vi "Drive Train Temps.vi"(8 "error in (no error)":errorcluster, 10 "Force Throttle?":bool, 11 "Falcon500 in":refnum<class "Falcon500.lvclass">) -> (0 "error out":errorcluster, 2 "Drive Train Tempuratures":T1, 3 "Falcon500 out":refnum<class "Falcon500.lvclass">)   [LabVIEW 2019, in "Drive.lvlib" / "Falcon500.lvclass"]
uses:
  Falcon500.lvclass
  C:/Users/Public/Documents/2020InfinteRecharge/src robot/Classes/Drive/Tank Drive/Tank Drive.lvclass
  Controls/Drive Train Temperatures.ctl
  <vilib>/Rock Robotics/WPI/ThirdParty/Phoenix-LabVIEW/Motor Controller/Controls/CTRE_Phoenix_MotorControl_StatorCurrentLimitConfiguration.ctl
  <vilib>/Rock Robotics/WPI/ThirdParty/Phoenix-LabVIEW/Motor Controller/Get/CTRE_Phoenix_MotorController_GetTemperature.vi
  <vilib>/Rock Robotics/Network Tables/NT Write Boolean.vi
  CTRE Drive.lvclass
  Tank Drive.lvclass
panel:
  out "Throttle?":bool
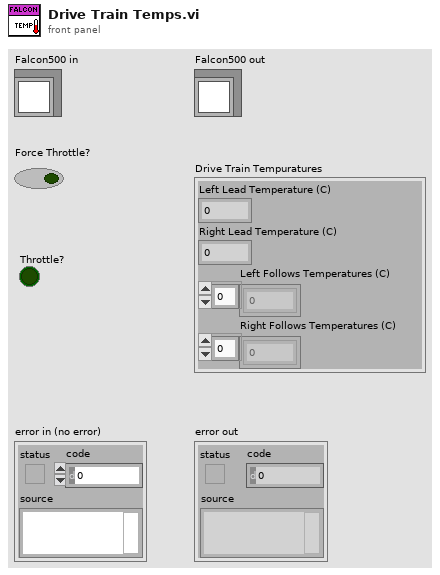
[diagram p1: front panel]
types:
  T1 = typedef "Drive.lvlib/Tank Drive.lvclass/Drive Train Temperatures.ctl" = cluster{"Left Lead Temperature (C)":dbl, "Right Lead Temperature (C)":dbl, "Left Follows Temperatures (C)":dbl[], "Right Follows Temperatures (C)":dbl[]}
  T2 = typedef "CTRE_Phoenix_MotorControl_StatorCurrentLimitConfiguration.ctl" = cluster{"Enable?":bool, "Current Limit":dbl, "Threshold Current":dbl, "Threshold Time":dbl}
  T3 = typedef "Drive.lvlib/Tank Drive.lvclass/Motor Controller Names.ctl" = cluster{"Left Lead":string, "Right Lead":string, "Left Followers":string[], "Right Followers":string[]}
  T4 = typedef "WPI_MotorControlDeviceRef.ctl" = cluster{"DeviceStatus":errorcluster, "Type":T5, "PWM":cluster{"PWM Channel":T6, "DeadBand":T7}, "CAN":cluster{"Device Number":u8, "SetOutput VI Ref":variant, "GetOutput VI Ref":variant, "Enable VI Ref":variant, "Disable VI Ref":variant, "Data":variant}, "Invert":bool, "DIO PWM":cluster{"PWM \"Enable\" Channel":T6, "DIOChannel":T8, "PWM Rate":dbl}}
  T5 = typedef "WPI_MotorControlType.ctl" = enum16{"PWM", "CAN", "DIO PWM"}
  T6 = typedef "FPGA_DIOPWMChannel.ctl" = enum8{"PWM 0", "PWM 1", "PWM 2", "PWM 3", "PWM 4", "PWM 5", "PWM 6", "PWM 7", "PWM 8", "PWM 9", "PWM MXP 0", "PWM MXP 1", "PWM MXP 2", "PWM MXP 3", "PWM MXP 4", "PWM MXP 5", "PWM MXP 6", "PWM MXP 7", "PWM MXP 8", "PWM MXP 9", "Invalid"}
  T7 = typedef "WPI_PWMDeadband.ctl" = cluster{"Name":string, "maxPositivePwm":i32, "minPositivePwm":i32, "centerPwm":i32, "maxNegativePwm":i32, "minNegativePwm":i32, "angularRange":u16}
  T8 = typedef "FPGA_DIOChannel.ctl" = enum8{"DIO 0", "DIO 1", "DIO 2", "DIO 3", "DIO 4", "DIO 5", "DIO 6", "DIO 7", "DIO 8", "DIO 9", "DIO MXP 0", "DIO MXP 1", "DIO MXP 2", "DIO MXP 3", "DIO MXP 4", "DIO MXP 5", "DIO MXP 6", "DIO MXP 7", "DIO MXP 8", "DIO MXP 9", "DIO MXP 10", "DIO MXP 11", "DIO MXP 12", "DIO MXP 13", "DIO MXP 14", "DIO MXP 15", "SPI Port CS1", "SPI Port CS2", "SPI Port CS3", "SPI Port MISO", "SPI Port MOSI", "Invalid"}
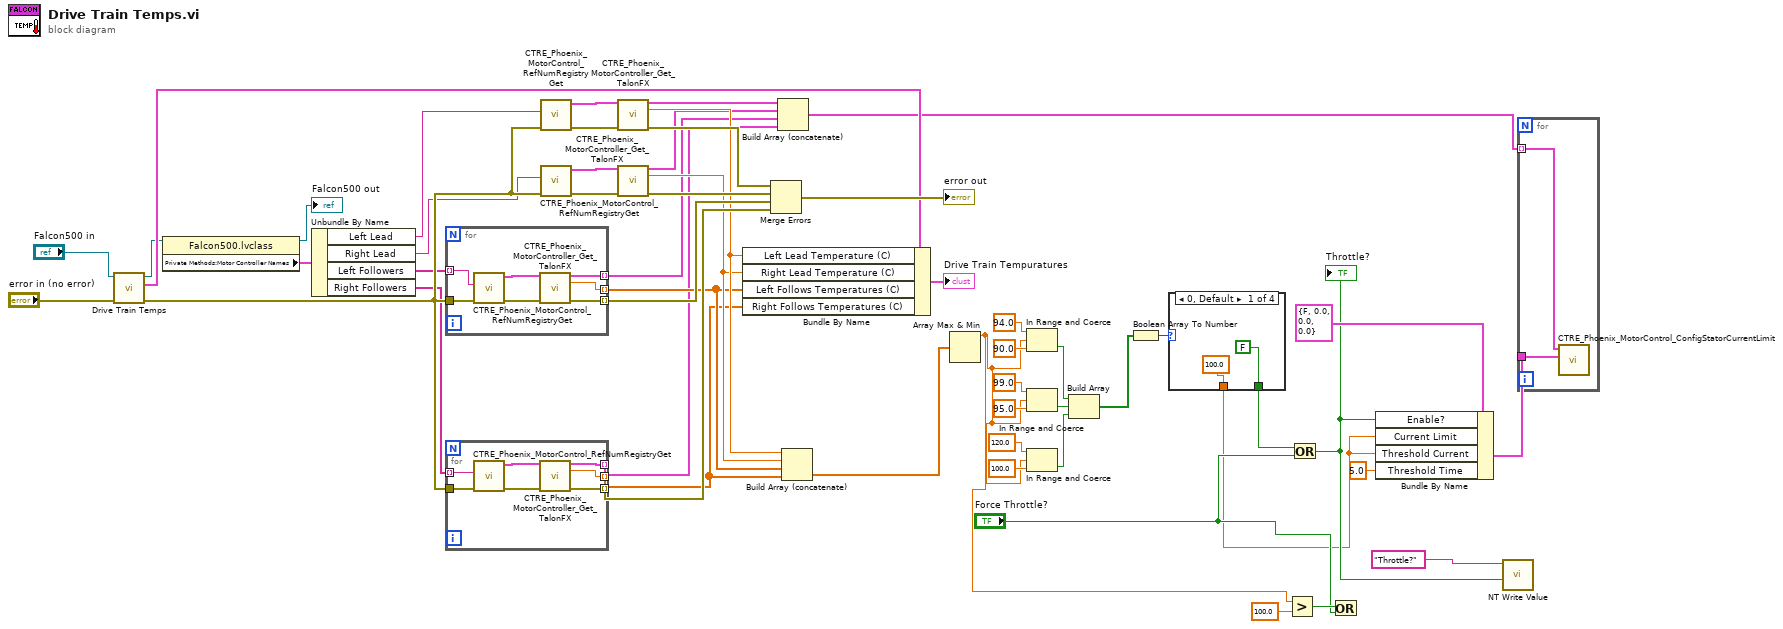
[diagram p0: block diagram]
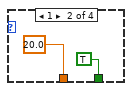
[diagram p2: hidden frame]
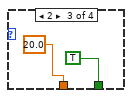
[diagram p3: hidden frame]
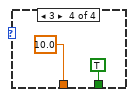
[diagram p4: hidden frame]
diagram:
  n1 = call-parent "Drive Train Temps.vi"("error in (no error)"="error in (no error)", "Tank Drive in"="Falcon500 in") -> ("error out"=w40:errorcluster, "Drive Train Temperatures"=w34:T1, "Tank Drive out"=w33:refnum<class "Falcon500.lvclass">)  [unwired: 7 in]
  n2 = property class="Falcon500.lvclass"(reference=w33) -> (reference out=→"Falcon500 out":refnum<class "Falcon500.lvclass">, "Private Methods:Motor Controller Names"=w52:T3)  [unwired: 1 in, 1 out]
  n3 = Unbundle By Name(w52) -> ("Left Lead"=w30:string, "Right Lead"=w29:string, "Left Followers"=w28:string[], "Right Followers"=w27:string[])
  n4 = for {
    tunnel: w28 -> [w58] mode=indexing
    tunnel: [w57] -> w37 mode=indexing
    tunnel: [w56] -> w44 mode=indexing
    tunnel: w40 -> [w55]
    tunnel: [w54] -> w22 mode=indexing
    n5 = call <vilib>:"CTRE_Phoenix_MotorControl_RefNumRegistryGet.vi"("error in (no error)"=w55, "refnum name"=w58) -> ("error out"=w59:errorcluster, "PhoenixMotorControlDevRef"=w60:T4)  [unwired: 8 in]
    n6 = call-poly <vilib>:"CTRE_Phoenix_MotorController_Get_TalonFX.vi"("PhoenixMotorControlDevRef"=w60, "error in"=w59) -> ("PhoenixMotorControlDevRef"=w54:T4, "Temperature (C)"=w57:dbl, "error out"=w56:errorcluster)  [unwired: 11 in]
  }
  n7 = for {
    tunnel: w27 -> [w65] mode=indexing
    tunnel: [w64] -> w36 mode=indexing
    tunnel: [w63] -> w43 mode=indexing
    tunnel: w40 -> [w62]
    tunnel: [w61] -> w21 mode=indexing
    n8 = call <vilib>:"CTRE_Phoenix_MotorControl_RefNumRegistryGet.vi"("error in (no error)"=w62, "refnum name"=w65) -> ("error out"=w67:errorcluster, "PhoenixMotorControlDevRef"=w66:T4)  [unwired: 8 in]
    n9 = call-poly <vilib>:"CTRE_Phoenix_MotorController_Get_TalonFX.vi"("PhoenixMotorControlDevRef"=w66, "error in"=w67) -> ("PhoenixMotorControlDevRef"=w61:T4, "Temperature (C)"=w64:dbl, "error out"=w63:errorcluster)  [unwired: 11 in]
  }
  n10 = call <vilib>:"CTRE_Phoenix_MotorControl_RefNumRegistryGet.vi"("error in (no error)"=w40, "refnum name"=w30) -> ("error out"=w50:errorcluster, "PhoenixMotorControlDevRef"=w51:T4)  [unwired: 8 in]
  n11 = call <vilib>:"CTRE_Phoenix_MotorControl_RefNumRegistryGet.vi"("error in (no error)"=w40, "refnum name"=w29) -> ("error out"=w49:errorcluster, "PhoenixMotorControlDevRef"=w48:T4)  [unwired: 8 in]
  n12 = call-poly <vilib>:"CTRE_Phoenix_MotorController_Get_TalonFX.vi"("PhoenixMotorControlDevRef"=w51, "error in"=w50) -> ("PhoenixMotorControlDevRef"=w25:T4, "Temperature (C)"=w39:dbl, "error out"=w46:errorcluster)  [unwired: 11 in]
  n13 = call-poly <vilib>:"CTRE_Phoenix_MotorController_Get_TalonFX.vi"("PhoenixMotorControlDevRef"=w48, "error in"=w49) -> ("PhoenixMotorControlDevRef"=w23:T4, "Temperature (C)"=w38:dbl, "error out"=w45:errorcluster)  [unwired: 11 in]
  n14 = Bundle By Name(cluster=w34, "Left Lead Temperature (C)"=w39, "Right Lead Temperature (C)"=w38, "Left Follows Temperatures (C)"=w37, "Right Follows Temperatures (C)"=w36) -> (→"Drive Train Tempuratures":T1)
  n15 = Merge Errors(w46, w45, w44, w43) -> (→"error out":errorcluster)
  n16 = Build Array (concatenate)(w25, w23, w22, w21) -> (w24:T4[])
  n17 = Build Array (concatenate)(w39, w38, w37, w36) -> (w35:dbl[])
  n18 = Array Max & Min(array=w35) -> (max value=w3:dbl)  [unwired: 3 out]
  n19 = In Range and Coerce(upper limit=94.0, x=w3, lower limit=90.0) -> (In Range?=w11:bool)  [unwired: 1 out]
  n20 = In Range and Coerce(upper limit=99.0, x=w3, lower limit=95.0) -> (In Range?=w8:bool)  [unwired: 1 out]
  n21 = In Range and Coerce(upper limit=120.0, x=w3, lower limit=100.0) -> (In Range?=w4:bool)  [unwired: 1 out]
  n22 = Build Array(w11, w8, w4) -> (w12:bool[])
  n23 = Boolean Array To Number(Boolean array=w12) -> (number=w7:u32)
  n24 = case shown="0, Default" w7 {
    tunnel: [FALSE ("x") TRUE ("x") TRUE ("x") TRUE ("x")] -> w2
    tunnel: [100.0 ("Current Limit") 20.0 ("Current Limit") 20.0 ("Current Limit") 10.0 ("Current Limit")] -> w1
    frame 0, Default {
    }
    frame 1 {
    }
    frame 2 {
    }
    frame 3 {
    }
  }
  n25 = Greater?(x=w3, y=100.0) -> (0:w17:bool)
  n26 = Or(x=w2, y="Force Throttle?") -> (x .or. y?=w19:bool)
  "Throttle?" <- w19
  n27 = Or(x=w17, y="Force Throttle?") -> ()  [unwired: 1 out]
  n28 = Bundle By Name(cluster=T2 {"Enable?"=FALSE, "Current Limit"=0.0, "Threshold Current"=0.0, "Threshold Time"=0.0} ("Stator Current Limit Configuration"), "Enable?"=w19, "Current Limit"=w1, "Threshold Current"=w1, "Threshold Time"=5.0) -> (w26:T2)
  n29 = call-poly <vilib>:"NT Write Value.vi"("Boolean"=w19, "Name"="Throttle?") -> ()  [unwired: 9 in, 1 out]
  n30 = for {
    tunnel: w26 -> [w77]
    tunnel: w24 -> [w76] mode=indexing
    n31 = call <vilib>:"CTRE_Phoenix_MotorControl_ConfigStatorCurrentLimit.vi"("Stator Current Limit Configuration"=w77, "PhoenixMotorControlDevRef"=w76) -> ()  [unwired: 8 in, 2 out]
  }
